vi "CmdExe.Wait then Launch App.vi"(10 "Delay(s)":i32=3, 11 "App Path":path=path "C:/Program Files (x86)/Valve/Test Executive/Test Executive.exe") -> ()   [LabVIEW 2018]
panel:
  out "StdErr":string
  out "StdOut":string
  out "Cmd":string
  out "error out":errorcluster
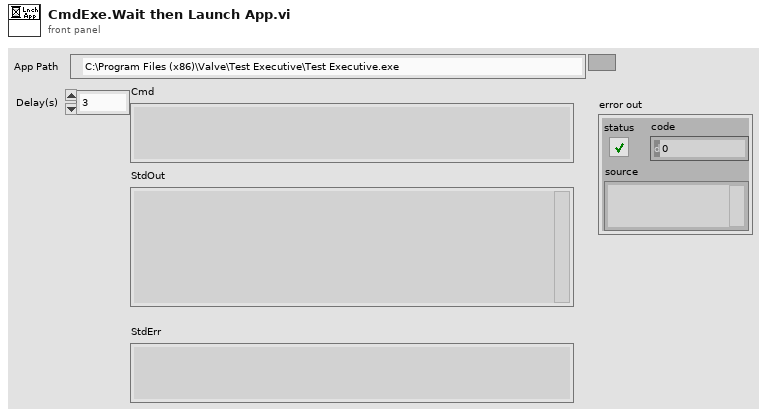
[diagram p1: front panel]
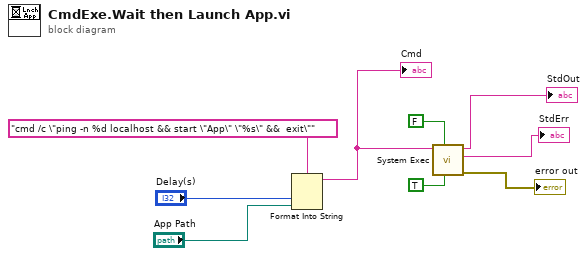
[diagram p0: block diagram]
diagram:
  n1 = Format Into String(format string="cmd /c \"ping -n %d localhost && start \"App\" \"%s\" &&  exit\"" ("command line"), "Delay(s)", "App Path") -> (resulting string=w1:string)  [unwired: 2 in, 1 out]
  "Cmd" <- w1
  n2 = call <vilib>:"System Exec.vi"("run minimized? (F)"=TRUE, "wait until completion? (T)"=FALSE, "command line"=w1) -> ("error out"=→"error out":errorcluster, "standard error"=→"StdErr":string, "standard output"=→"StdOut":string)  [unwired: 5 in, 1 out]
